vi "Daemon_CreateStore.vi"(7 "Dialog Name":string, 10 "Dialog Parameters":string, 11 "jModule":refnum<class "jModule.lvclass">) -> ()   [LabVIEW 2020]
doc: "created using\nJSMA Daemon Template - Two Button Prompt 0.2.0.2\nRob Humfeld - Jet Engineering\nCopyright (c) 2020, Jet Engineering"
uses:
  Daemon_CreateStore - Status STYP.ctl
  <userlib>/JET Engineering/JSMA/Libraries/jModule Class/jModule.lvclass
  <userlib>/Jet Labs/JET Panel/JETPanel_Behavior_STYP.ctl
  <userlib>/JET Engineering/JET_QSM/Code/Private/JET_QSM - Add State [String API].vi
  <userlib>/JET Engineering/JSMA/Libraries/jModule Class/Read RxQueue.vi
  <vilib>/Utility/error.llb/Trim Whitespace.vi
  <vilib>/Utility/error.llb/Error Cluster From Error Code.vi
  <userlib>/JET Engineering/JSMA/Libraries/jMsg Class/jMsg.lvclass
  <userlib>/JET Labs/JET Panel/JETPanel.lvclass
panel:
  out "Prompt":string
  in  "OK Button":bool
  in  "Cancel Button":bool
  out "winSizer 2":string="W"
  out "winSizer 1":string="W"
  out "Recent states before Error (with tick counts) 2":string
  in  "Status":T1
  out "error out":errorcluster
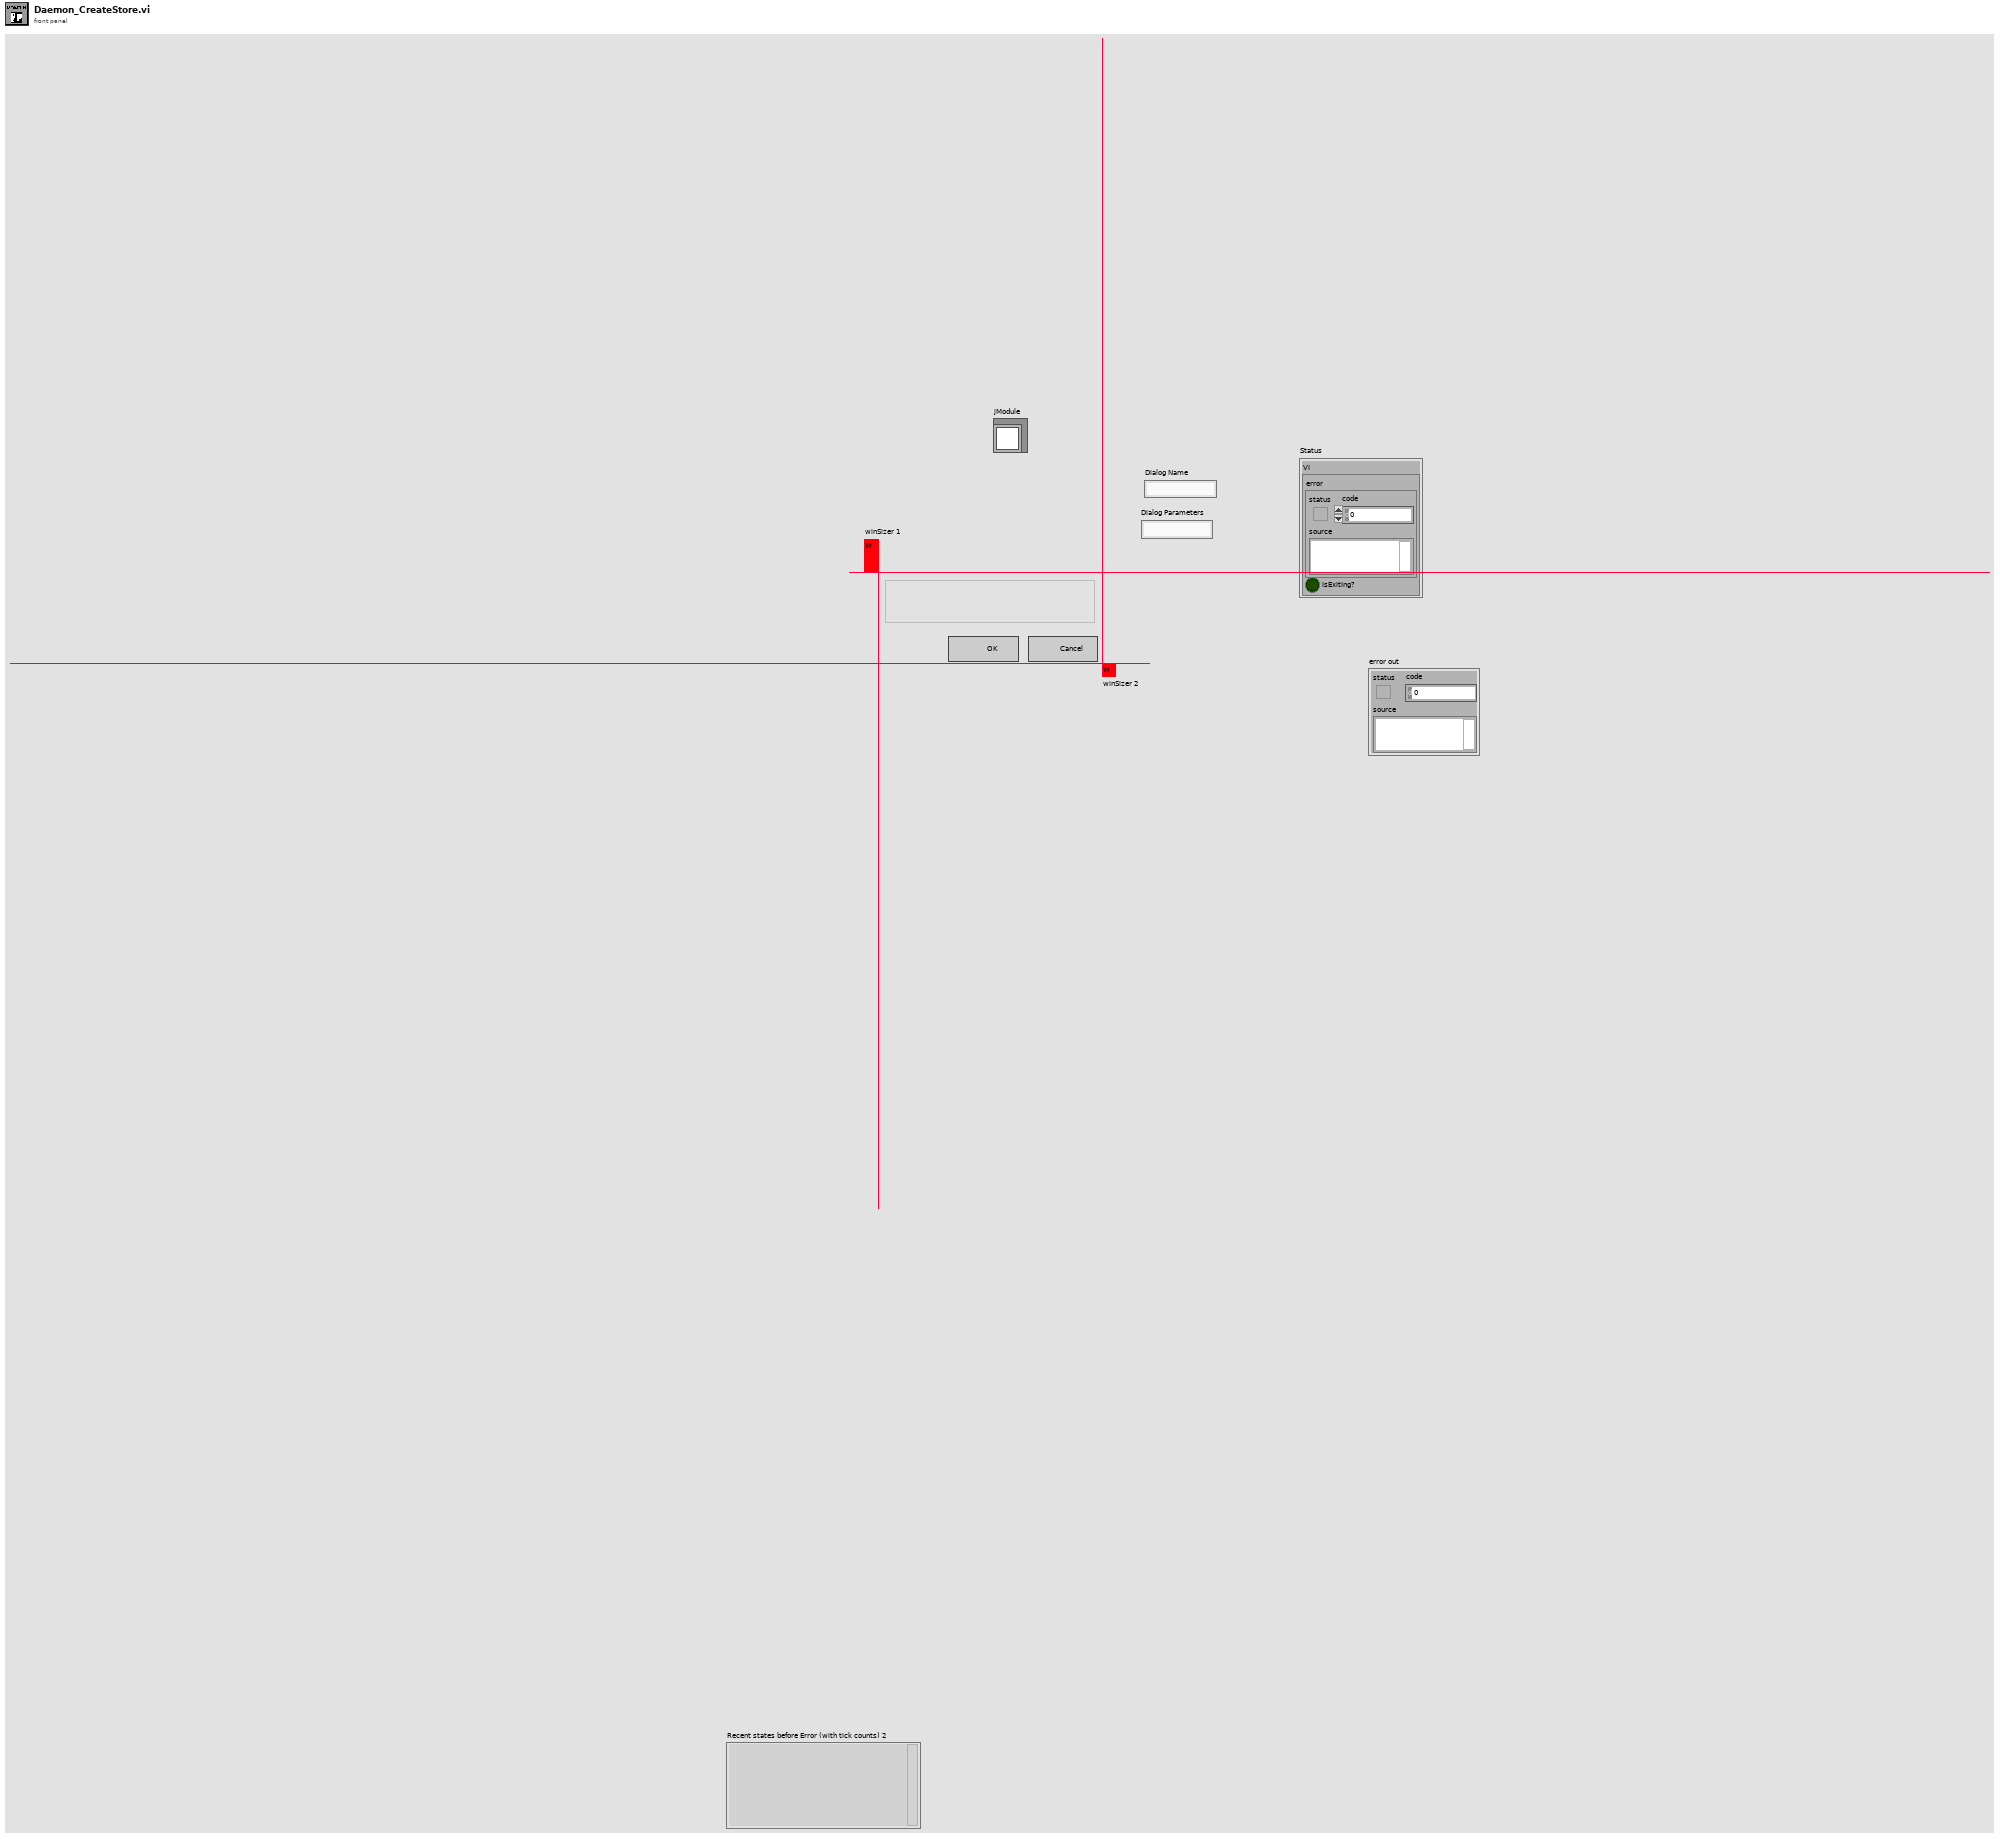
[diagram p1: front panel]
types:
  T1 = typedef "Daemon_CreateStore - Status STYP.ctl" = cluster{"VI":cluster{"error":errorcluster, "isExiting?":bool}}
  T2 = typedef "JETPanel_Behavior_STYP.ctl" = enum32{"Default", "Modal", "Floating", "Floating/Auto-Hide"}
  T3 = typedef "JET_QSM_Refnum STYP.ctl" = cluster{"state":cluster{"queue":refnum<queue>, "idle":string, "error":string, "STOP":string}, "debug":cluster{"enabled?":bool, "queue":refnum<queue>}, "Invalid.option":T4, "QSM.Name":string}
  T4 = typedef "JET_QSM_InvalidOption STYP.ctl" = enum16{"Ignore", "Dialog", "Error"}
  T5 = typedef "JET_QSM_Element STYP.ctl" = cluster{"state":string, "data":variant, "comment":string}
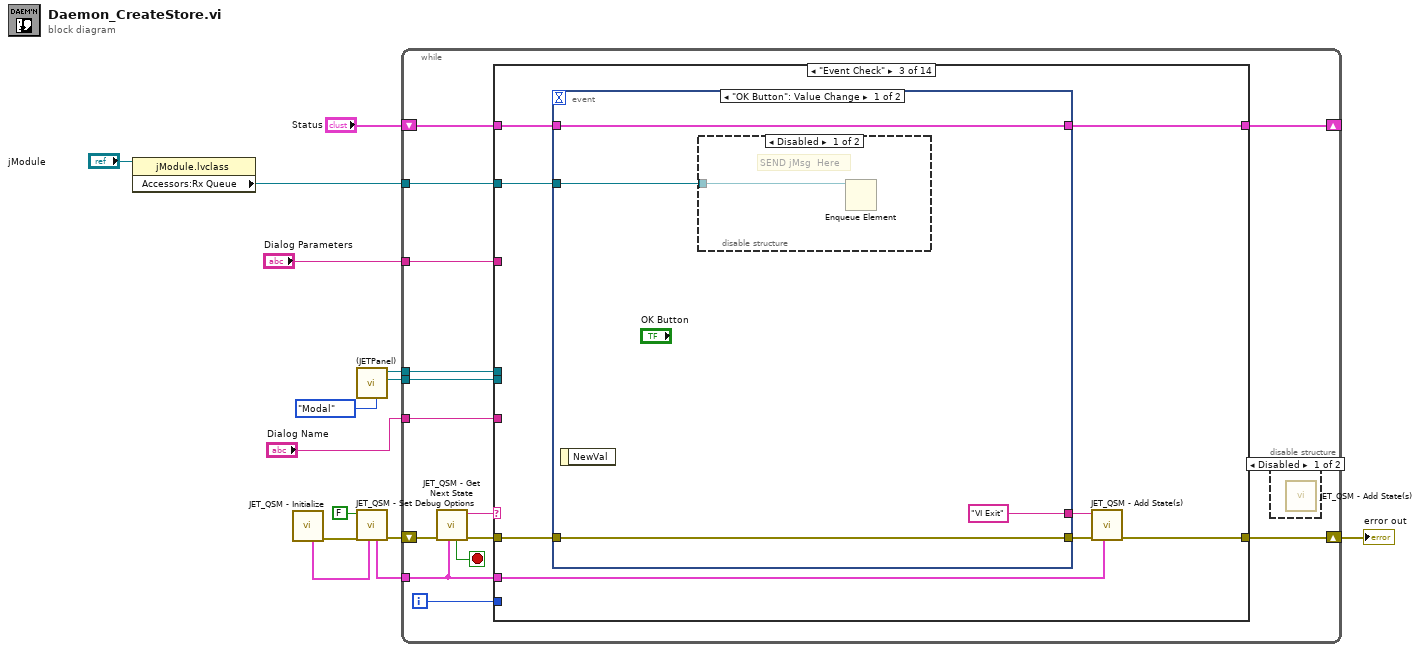
[diagram p0: block diagram]
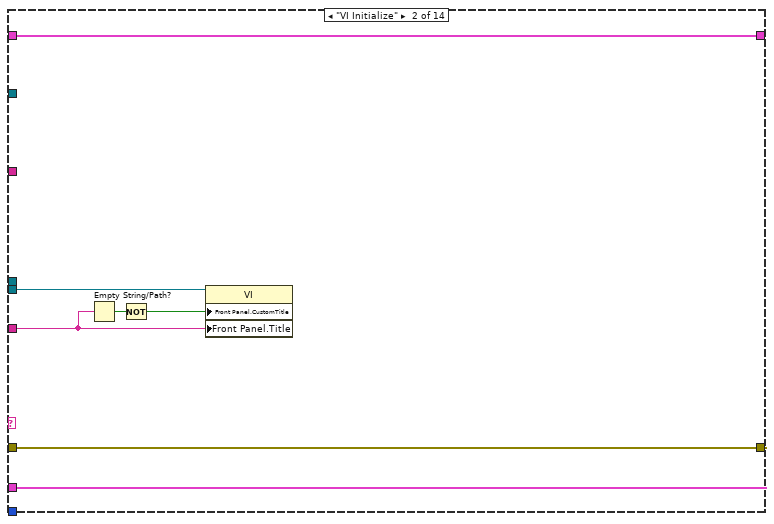
[diagram p4: hidden frame]
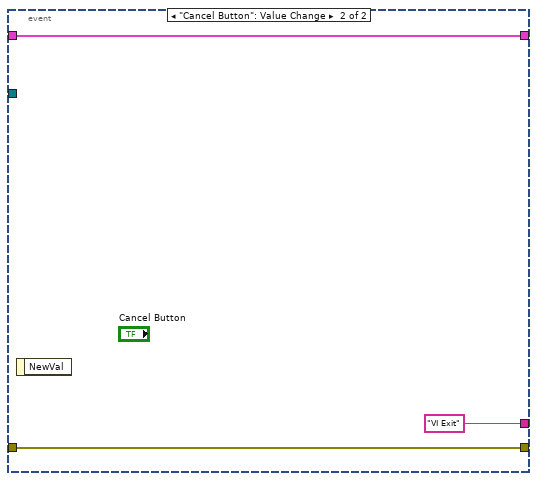
[diagram p6: hidden frame]
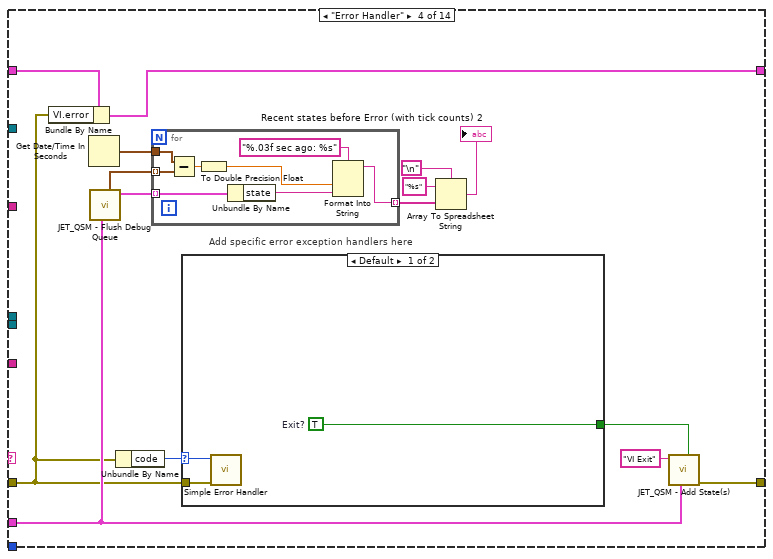
[diagram p7: hidden frame]
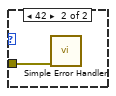
[diagram p8: hidden frame]
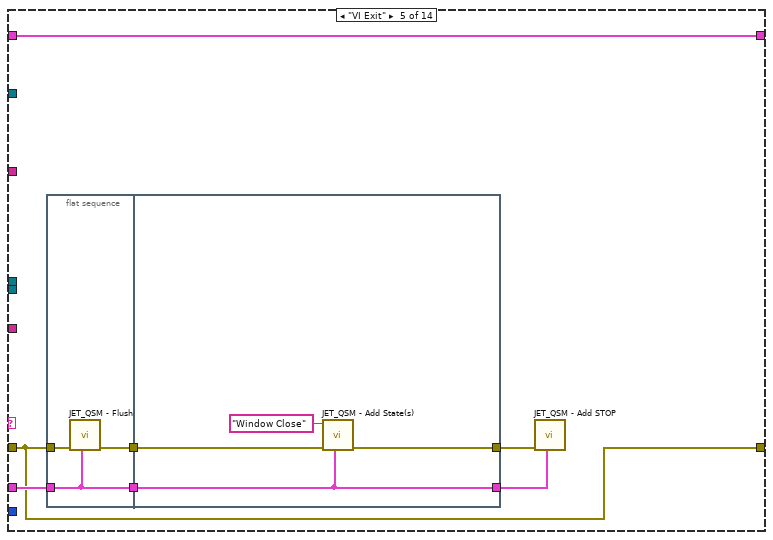
[diagram p9: hidden frame]
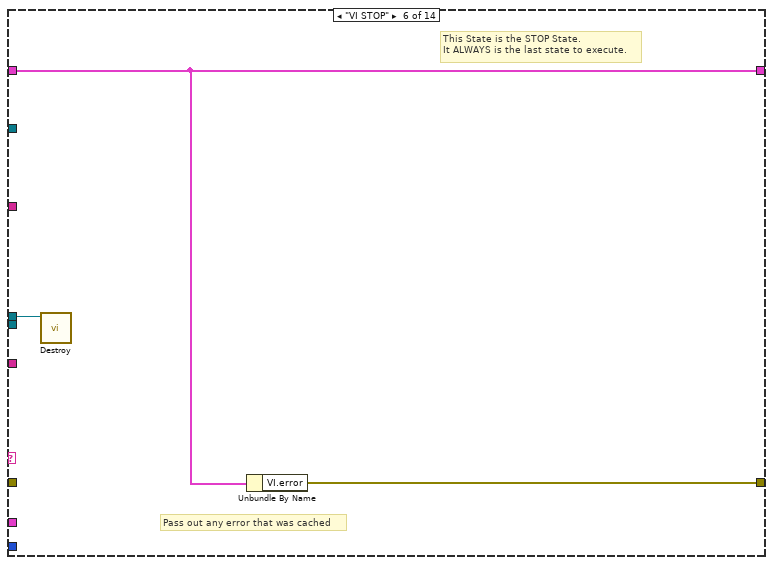
[diagram p10: hidden frame]
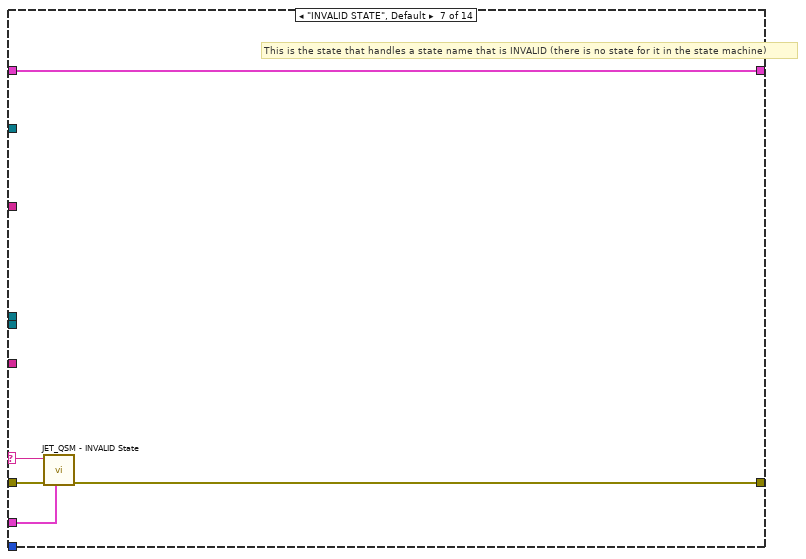
[diagram p11: hidden frame]
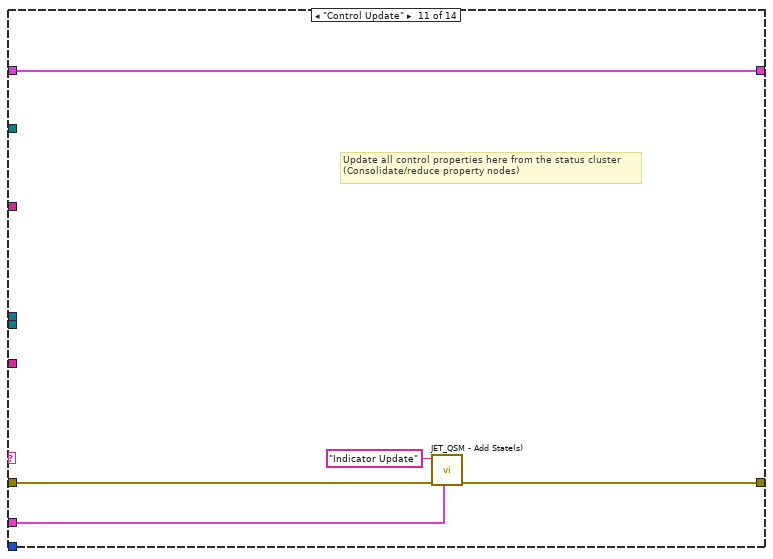
[diagram p15: hidden frame]
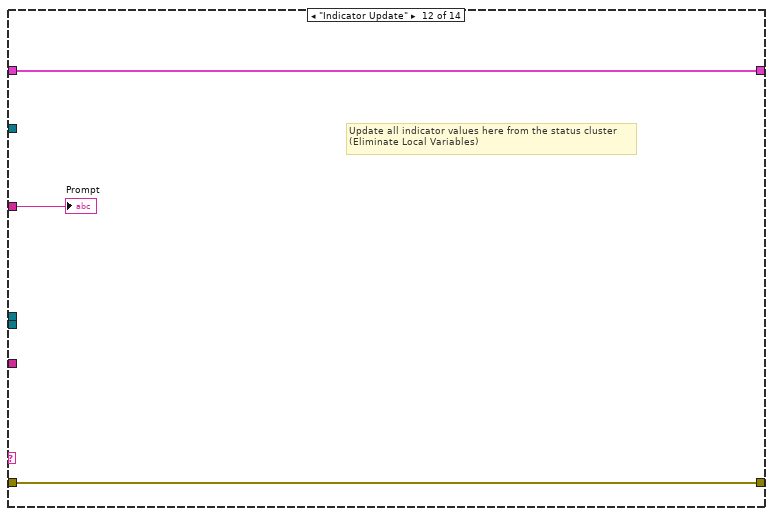
[diagram p16: hidden frame]
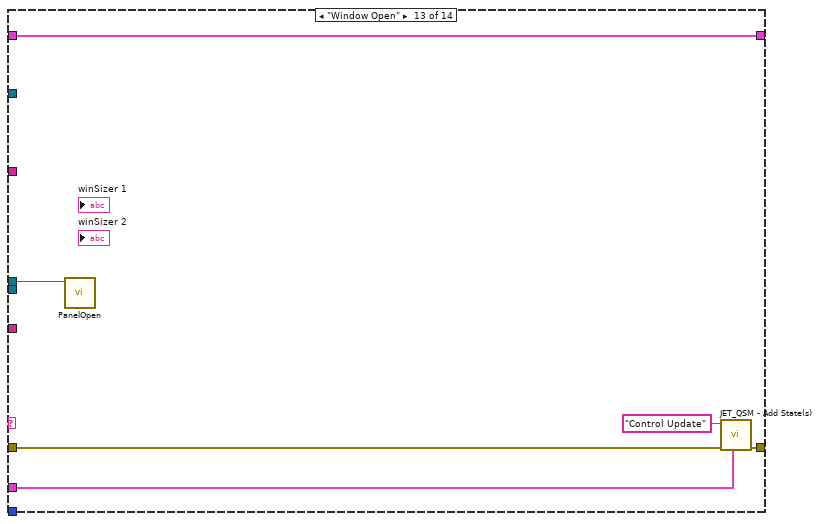
[diagram p17: hidden frame]
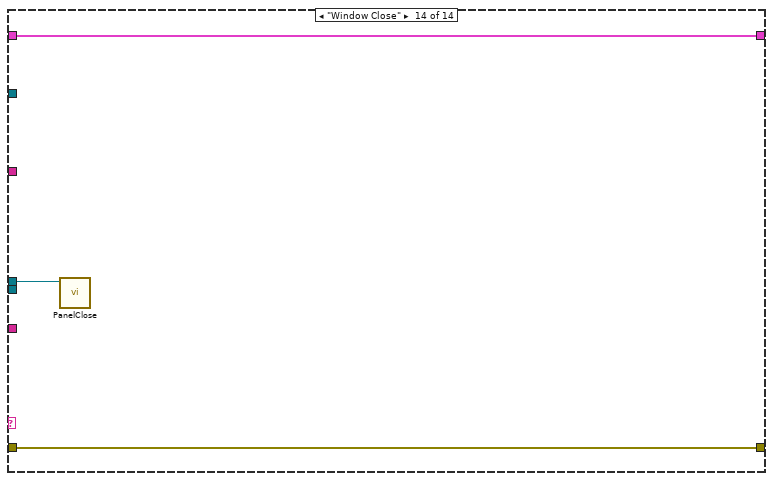
[diagram p18: hidden frame]
diagram:
  n1 = property class="jModule.lvclass"(reference="jModule") -> ("Accessors:Rx Queue"=w1:refnum<queue>)  [unwired: 1 in, 2 out]
  n2 = call <userlib>:"JET_QSM - Initialize.vi"() -> ("error out"=w14:errorcluster, "Jet_QSM refnum"=w11:T3)  [unwired: 10 in]
  n3 = call <userlib>:"(JETPanel).vi"("Behavior (Default)"=JETPanel_Behavior_STYP."Modal") -> ("VI Refnum"=w4:refnum<vi>, "JETPanel"=w6:refnum<class "JETPanel.lvclass">)  [unwired: 7 in, 2 out]
  n4 = call <userlib>:"JET_QSM - Set Debug Options.vi"("Jet_QSM refnum"=w11, "error in (no error)"=w14, "debug.enabled? (F)"=FALSE) -> ("error out"=w13:errorcluster, "Jet_QSM ref"=w12:T3)  [unwired: 7 in]
  n5 = while {
    tunnel: w12 -> [w24]
    shift-right: [w22] -> _
    shift-left: "Status" -> [w23]
    shift-right: [w21] -> w8
    shift-left: w13 -> [w28]
    tunnel: w6 -> [w19]
    tunnel: "Dialog Parameters" -> [w18]
    tunnel: w4 -> [w17]
    tunnel: "Dialog Name" -> [w16]
    tunnel: w1 -> [w15]
    i -> [w20]
    stop <- w25 stop-if-true
    n6 = call <userlib>:"JET_QSM - Get Next State.vi"("Jet_QSM refnum"=w24, "error in (no error)"=w28) -> ("error out"=w27:errorcluster, "state"=w26:string, "Stop Loop?"=w25:bool)  [unwired: 5 in, 2 out]
    n7 = case shown="\"Event Check\"" w26 {
      selector: w26 -> [_ _ _ _ _ _ w102 _ _ _ _ _ _ _]
      tunnel: w27 -> [w29 w39 w44 w58 w83 _ w103 w105 w107 w109 w112 w117 w121 w126]
      tunnel: w24 -> [_ w37 w47 w62 w88 _ w101 _ _ _ w113 _ w122 _]
      tunnel: w23 -> [w30 w35 w46 w57 w86 w98 w104 w106 w108 w110 w115 w118 w124 w127]
      tunnel: [w30 w35 w45 w56 w86 w98 w104 w106 w108 w110 w115 w118 w124 w127] -> w22
      tunnel: [w29 w36 w42 w63 w83 w99 w100 w105 w107 w109 w111 w117 w120 w126] -> w21
      tunnel: w20 -> [_ _ _ _ _ _ _ _ _ _ _ _ _ _]
      tunnel: w19 -> [_ _ _ _ _ w97 _ _ _ _ _ _ w119 w125]
      tunnel: w18 -> [_ _ _ _ _ _ _ _ _ _ _ w116 _ _]
      tunnel: w17 -> [_ w34 _ _ _ _ _ _ _ _ _ _ _ _]
      tunnel: w16 -> [_ w33 _ _ _ _ _ _ _ _ _ _ _ _]
      tunnel: w15 -> [_ _ w40 _ _ _ _ _ _ _ _ _ _ _]
      frame "------ Standard States ------" {
        # "Standard States are required states for a JET_QSM State Machine\n\nTheir names may be changed; use the Initialize function to specify the new names"
        # "This is a section header; the state is never expected to execute"
      }
      frame "VI Initialize" {
        n8 = Empty String/Path?(string/path=w33) -> (empty?=w32:bool)
        n9 = Not(x=w32) -> (.not. x?=w31:bool)
        n10 = property class="VI"(reference=w34, "Front Panel.CustomTitle"=w31, "Front Panel.Title"=w33) -> ()  [unwired: 1 in, 2 out]
        n11 = call-poly <userlib>:"JET_QSM - Add State(s).vi"("Jet_QSM refnum"=w37, "error in (no error)"=w39, "state(s)"="Window Open") -> ("error out"=w36:errorcluster)  [unwired: 8 in]
      }
      frame "Event Check" {
        n12 = event shown="[0] \"OK Button\": Value Change" {
          selector: _ -> [_ _]
          dyn-events: _ -> [_ _]
          timeout: _ -> [_ _]
          tunnel: w46 -> [w51 w55]
          tunnel: [w51 w55] -> w45
          tunnel: w44 -> [w50 w54]
          tunnel: [w50 w54] -> w43
          tunnel: ["VI Exit" ("state(s)") "VI Exit" ("state(s)")] -> w41
          tunnel: w40 -> [w48 _]
          event "OK Button": Value Change {
            n13 = event-data() -> ()  [unwired: 1 in, 1 out]
            n14 = disable-structure shown="Disabled" {
              disable-tunnel: w48 -> [w52 _]
              frame Disabled {
                # "SEND jMsg  Here"
                n15 = Enqueue Element(queue=w52) -> ()  [unwired: 3 in, 3 out]
              }
              frame Enabled {
              }
            }
          }
          event "Cancel Button": Value Change {
            n16 = event-data() -> ()  [unwired: 1 in, 1 out]
          }
        }
        n17 = call-poly <userlib>:"JET_QSM - Add State(s).vi"("Jet_QSM refnum"=w47, "error in (no error)"=w43, "state(s)"=w41) -> ("error out"=w42:errorcluster)  [unwired: 8 in]
      }
      frame "Error Handler" {
        # "Add specific error exception handlers here"
        n18 = Bundle By Name(cluster=w57, "VI.error"=w58) -> (w56:T1)
        n19 = Get Date/Time In Seconds() -> (seconds since 1Jan1904=w66:timestamp)
        n20 = call <userlib>:"JET_QSM - Flush Debug Queue.vi"("Jet_QSM refnum"=w62) -> ("QSM Elements"=w64:T5[], "Timestamps"=w65:timestamp[])  [unwired: 8 in, 1 out]
        n21 = Unbundle By Name(w58) -> ("code"=w59:i32)
        n22 = for {
          tunnel: w64 -> [w78] mode=indexing
          tunnel: [w76] -> w68 mode=indexing
          tunnel: w66 -> [w73]
          tunnel: w65 -> [w74] mode=indexing
          n23 = Subtract(x=w73, y=w74) -> (x-y=w72:dbl)
          n24 = To Double Precision Float(number=w72) -> (double precision float=w71:dbl)
          n25 = Unbundle By Name(w78) -> ("state"=w77:string)
          n26 = Format Into String(format string="%.03f sec ago: %s", w71, w77) -> (resulting string=w76:string)  [unwired: 2 in, 1 out]
        }
        n27 = case shown="Default" w59 {
          selector: w59 -> [w80 _]
          tunnel: [w81 _] -> w60
          tunnel: w58 -> [w79 w82]
          frame Default {
            w81 = TRUE  # Exit?
            n28 = call <vilib>:"Simple Error Handler.vi"("error code (no error:0)"=w80, "error in (no error)"=w79) -> ()  [unwired: 3 in, 5 out]
          }
          frame 42 {
            n29 = call <vilib>:"Simple Error Handler.vi"("error in (no error)"=w82) -> ()  [unwired: 4 in, 5 out]
          }
        }
        n30 = Array To Spreadsheet String(delimiter (Tab)="\n", array=w68, 3:"%s" ("format string")) -> (spreadsheet string=→"Recent states before Error (with tick counts) 2":string)
        n31 = call-poly <userlib>:"JET_QSM - Add State(s).vi"("act? (T)"=w60, "Jet_QSM refnum"=w62, "state(s)"="VI Exit") -> ("error out"=w63:errorcluster)  [unwired: 8 in]
      }
      frame "VI Exit" {
        n32 = flat-sequence {
          tunnel: w83 -> [w92]
          tunnel: w88 -> [w90]
          tunnel: [w91] -> w85
          tunnel: [w90] -> w84
          tunnel: [w96] -> w87
          tunnel: [w93] -> w89
          tunnel: w85 -> [w94]
          tunnel: w84 -> [w96]
          frame #0 {
            n33 = call <userlib>:"JET_QSM - Flush.vi"("Jet_QSM ref"=w90, "error in (no error)"=w92) -> ("error out"=w91:errorcluster)  [unwired: 8 in, 1 out]
          }
          frame #1 {
            n34 = call-poly <userlib>:"JET_QSM - Add State(s).vi"("Jet_QSM refnum"=w96, "error in (no error)"=w94, "state(s)"="Window Close") -> ("error out"=w93:errorcluster)  [unwired: 8 in]
          }
        }
        n35 = call <userlib>:"JET_QSM - Add STOP.vi"("Jet_QSM refnum"=w87, "error in (no error)"=w89) -> ()  [unwired: 9 in, 1 out]
      }
      frame "VI STOP" {
        # "Pass out any error that was cached"
        # "This State is the STOP State.\nIt ALWAYS is the last state to execute."
        n36 = call-dynamic "Destroy.vi"("JETPanel in"=w97) -> ()  [unwired: 10 in, 1 out]
        n37 = Unbundle By Name(w98) -> ("VI.error"=w99:errorcluster)
      }
      frame "INVALID STATE", Default {
        # "This is the state that handles a state name that is INVALID (there is no state for it in the state machine)"
        n38 = call <userlib>:"JET_QSM - INVALID State.vi"("Jet_QSM refnum"=w101, "error in (no error)"=w103, "state"=w102) -> ("error out"=w100:errorcluster)  [unwired: 8 in]
      }
      frame "------ Menu Commands ------" {
        # "This is a section header; the state is never expected to execute"
      }
      frame "------ Actions  ------" {
        # "This is a section header; the state is never expected to execute"
      }
      frame "------ Window and Panel Control ------" {
        # "This is a section header; the state is never expected to execute"
      }
      frame "Control Update" {
        # "Update all control properties here from the status cluster\n(Consolidate/reduce property nodes)"
        n39 = call-poly <userlib>:"JET_QSM - Add State(s).vi"("Jet_QSM refnum"=w113, "error in (no error)"=w112, "state(s)"="Indicator Update") -> ("error out"=w111:errorcluster)  [unwired: 8 in]
      }
      frame "Indicator Update" {
        # "Update all indicator values here from the status cluster\n(Eliminate Local Variables)"
        "Prompt" <- w116
      }
      frame "Window Open" {
        n40 = call-dynamic "PanelOpen.vi"("JETPanel in"=w119) -> ()  [unwired: 9 in, 2 out]
        n41 = call-poly <userlib>:"JET_QSM - Add State(s).vi"("Jet_QSM refnum"=w122, "error in (no error)"=w121, "state(s)"="Control Update") -> ("error out"=w120:errorcluster)  [unwired: 8 in]
      }
      frame "Window Close" {
        n42 = call-dynamic "PanelClose.vi"("JETPanel"=w125) -> ()  [unwired: 9 in, 2 out]
      }
    }
    n43 = disable-structure shown="Disabled" {
      frame Disabled {
        n44 = call-poly <userlib>:"JET_QSM - Add State(s).vi"() -> ()  [unwired: 11 in, 1 out]
      }
      frame Enabled {
      }
    }
  }
  "error out" <- w8
